vi "nPr.vi"(1 "R":i32, 2 "N":i32) -> (0 "Combinations":i32)   [LabVIEW 2010]
uses:
  <vilib>/gmath/NI_Gmath.lvlib
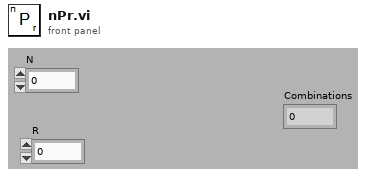
[diagram p1: front panel]
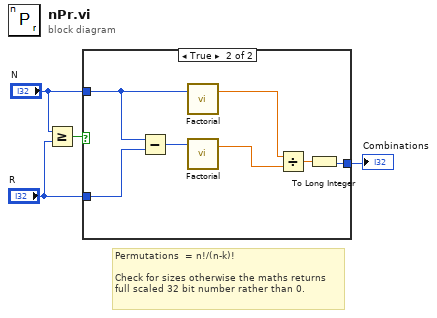
[diagram p0: block diagram]
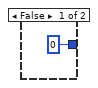
[diagram p2: hidden frame]
diagram:
  # "Permutations  = n!/(n-k)!\n\nCheck for sizes otherwise the maths returns\nfull scaled 32 bit number rather than 0."
  n1 = Greater Or Equal?(x="N", y="R") -> (x >= y?=w3:bool)
  n2 = case shown="True" w3 {
    tunnel: "N" -> [_ w12]
    tunnel: "R" -> [_ w11]
    tunnel: [0 w7] -> w4
    frame False {
    }
    frame True {
      n3 = Subtract(x=w12, y=w11) -> (x-y=w10:i32)
      n4 = call <vilib>:"Factorial.vi"("n"=w12) -> ("n!"=w9:dbl)  [unwired: 2 in]
      n5 = call <vilib>:"Factorial.vi"("n"=w10) -> ("n!"=w6:dbl)  [unwired: 2 in]
      n6 = Divide(x=w9, y=w6) -> (x/y=w8:dbl)
      n7 = To Long Integer(number=w8) -> (32bit integer=w7:i32)
    }
  }
  "Combinations" <- w4
